vi "SubtractRings1D.vi"(2 "delay pts inner":i32, 3 "delay pts outer":i32, 4 "h(r,t) ring inner":dbl[](array[numeric]) format="%.2f", 5 "h(r,t) ring outer":dbl[](array[numeric]) format="%.2f") -> (0 "delay pts out":i32, 1 "h(r,t) annulus":dbl[](array[numeric]) format="%.2f")   [LabVIEW 2022 SP3]
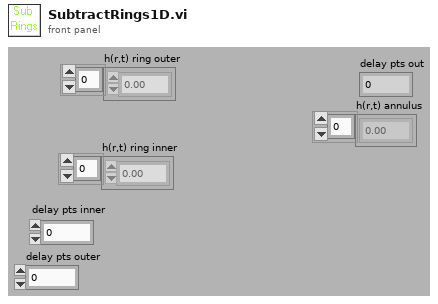
[diagram p1: front panel]
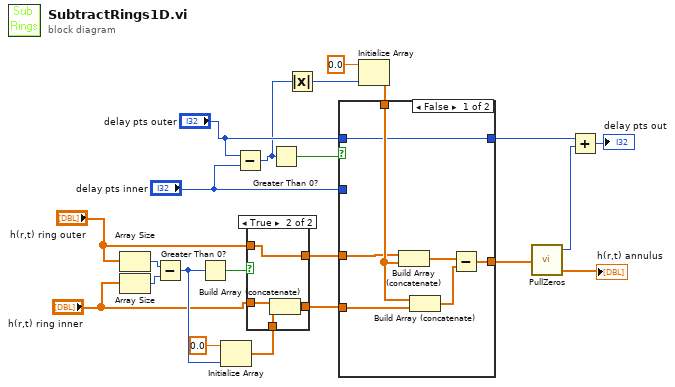
[diagram p0: block diagram]
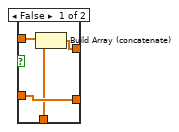
[diagram p2: hidden frame]
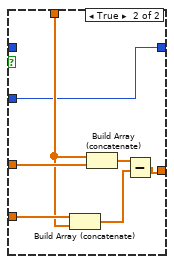
[diagram p3: hidden frame]
diagram:
  n1 = Array Size(array="h(r,t) ring outer") -> (size(s)=w10:i32)
  n2 = Array Size(array="h(r,t) ring inner") -> (size(s)=w9:i32)
  n3 = Subtract(x=w10, y=w9) -> (x-y=w7:i32)
  n4 = Greater Than 0?(x=w7) -> (x > 0?=w6:bool)
  n5 = Initialize Array(0.0, w7) -> (w4:dbl[])
  n6 = Subtract(x="delay pts outer", y="delay pts inner") -> (x-y=w13:i32)
  n7 = case shown="True" w6 {
    tunnel: "h(r,t) ring inner" -> [w26 w30]
    tunnel: w4 -> [w23 w29]
    tunnel: [w26 w28] -> w3
    tunnel: "h(r,t) ring outer" -> [w25 w27]
    tunnel: [w24 w27] -> w1
    frame False {
      n8 = Build Array (concatenate)(w25, w23) -> (w24:dbl[])
    }
    frame True {
      n9 = Build Array (concatenate)(w30, w29) -> (w28:dbl[])
    }
  }
  n10 = Greater Than 0?(x=w13) -> (x > 0?=w14:bool)
  n11 = Absolute Value(x=w13) -> (abs(x)=w12:i32)
  n12 = Initialize Array(0.0, w12) -> (w20:dbl[])
  n13 = case shown="False" w14 {
    tunnel: w1 -> [w32 w44]
    tunnel: w3 -> [w31 w42]
    tunnel: w20 -> [w36 w41]
    tunnel: [w37 w43] -> w11
    tunnel: "delay pts inner" -> [_ w38]
    tunnel: "delay pts outer" -> [w33 _]
    tunnel: [w33 w38] -> w18
    frame False {
      n14 = Build Array (concatenate)(w32, w36) -> (w35:dbl[])
      n15 = Build Array (concatenate)(w36, w31) -> (w34:dbl[])
      n16 = Subtract(x=w35, y=w34) -> (x-y=w37:dbl[])
    }
    frame True {
      n17 = Build Array (concatenate)(w42, w41) -> (w39:dbl[])
      n18 = Build Array (concatenate)(w41, w44) -> (w40:dbl[])
      n19 = Subtract(x=w40, y=w39) -> (x-y=w43:dbl[])
    }
  }
  n20 = call "PullZeros.vi"("input"=w11) -> ("output"=→"h(r,t) annulus":dbl[], "pre-zeros"=w19:i32)  [unwired: 3 out]
  n21 = Add(x=w18, y=w19) -> (x+y=→"delay pts out":i32)
